vi "launch_timer.vi"(8 "error in (no error)":errorcluster, 9 "Message Queues in":T2, 11 "test mode in":T1(ring)) -> (0 "error out":errorcluster, 1 "Message Queues out":T2, 3 "test mode out":T1(ring))   [LabVIEW 2015]
uses:
  support/Message Queue/All Message Queues.ctl
  support/Message Queue/Message Cluster.ctl
  support/Message Queue/Enqueue Message (Array).vi
  support/Message Queue/Message Queue.lvlib
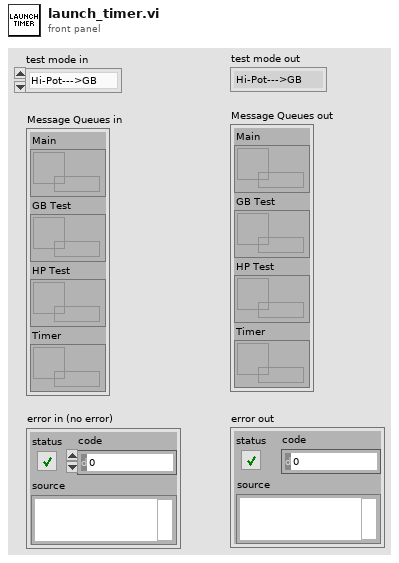
[diagram p1: front panel]
types:
  T1 = enum16{"Hi-Pot--->GB", "GB--->Hi-Pot", "Hi-Pot only", "GB only"}
  T2 = typedef "Message Queue.lvlib/All Message Queues.ctl" = cluster{"Main":refnum<queue>, "GB Test":refnum<queue>, "HP Test":refnum<queue>, "Timer":refnum<queue>}
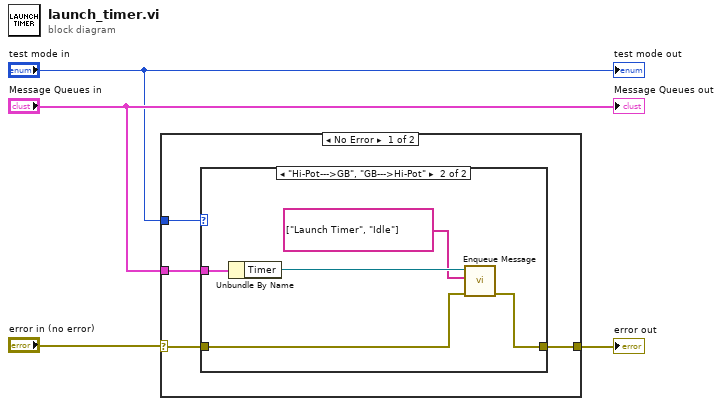
[diagram p0: block diagram]
diagram:
  n1 = case shown="No Error" "error in (no error)" {
    selector: "error in (no error)" -> [w6 w15]
    tunnel: "Message Queues in" -> [w8 _]
    tunnel: [w7 w15] -> w4
    tunnel: "test mode in" -> [w5 _]
    frame No Error {
      n2 = case shown="\"Hi-Pot--->GB\", \"GB--->Hi-Pot\"" w5 {
        tunnel: w8 -> [_ w14]
        tunnel: [w9 w13] -> w7
        tunnel: w6 -> [w9 w10]
        frame "Hi-Pot only", "GB only" {
        }
        frame "Hi-Pot--->GB", "GB--->Hi-Pot" {
          n3 = Unbundle By Name(w14) -> ("Timer"=w12:refnum<queue>)
          n4 = call-poly "Enqueue Message.vi"("error in (no error)"=w10, "Message Array"=string[] ["Launch Timer", "Idle"], "Message Queue"=w12) -> ("error out"=w13:errorcluster)  [unwired: 7 in, 1 out]
        }
      }
    }
    frame Error {
    }
  }
  "error out" <- w4
  "Message Queues out" <- "Message Queues in"
  "test mode out" <- "test mode in"
